vi "Test Basic Messaging.vi"(8 "error in":errorcluster, 11 "Test Case In":refnum<class "Messaging Tests.lvclass">) -> (0 "error out":errorcluster, 3 "Test Case Out":refnum<class "Messaging Tests.lvclass">)   [LabVIEW 2020, in "Messaging Tests.lvlib" / "Messaging Tests.lvclass"]
uses:
  Messaging Tests.lvclass
  C:/Program Files/National Instruments/LabVIEW 2024/vi.lib/Astemes/LUnit/Test Case.lvclass
  TestActor/TestActor.lvclass
  C:/Users/J63553/Projects/_LabVIEW Community/actor-framework/Core/ActorFramework/Actor/Actor.lvclass
  Core/ActorFramework/LastAck/Last Ack.lvclass
  Core/ActorFramework/Message Queue/Message Queue.lvclass/Message Queue.ctl
  Increment Msg/Increment Msg.lvclass/Increment Msg.ctl
  Core/ActorFramework/Message Enqueuer/Message Enqueuer.lvclass/Message Enqueuer.ctl
  Core/ActorFramework/Message Dequeuer/Message Dequeuer.lvclass/Message Dequeuer.ctl
  Core/ActorFramework/LastAck/Last Ack.lvclass/Last Ack.ctl
  TestActor/TestActor.lvclass/TestActor.ctl
  <vilib>/Astemes/LUnit/Test Case.lvclass/Test Case.ctl
  4635b618-f356-4e6f-9d02-cf2597439e9c.vi
  40d5848f-1082-4b1b-baa8-dc5717502d9b.vi
  <vilib>/Astemes/LUnit/Append Pass Result.vi
  <vilib>/Astemes/LUnit/Append Fail Result.vi
  4635b618-f356-4e6f-9d02-cf2597439e9c.vi/9c5d11cd-9439-4240-a1ee-d9baace9c924.vi
  40d5848f-1082-4b1b-baa8-dc5717502d9b.vi/9c5d11cd-9439-4240-a1ee-d9baace9c924.vi
  Core/ActorFramework/Message Enqueuer/Enqueue.vi
  <vilib>/Astemes/LUnit/Run In UI.vi
  <vilib>/Utility/error.llb/Clear Errors.vi
  Increment Msg/Increment Msg.lvclass
  C:/Users/J63553/Projects/_LabVIEW Community/actor-framework/Core/ActorFramework/Message/Message.lvclass
  Core/ActorFramework/Stop Msg/Stop Msg.lvclass
  Core/ActorFramework/Message Priority Queue/Priority Dequeue.vi
  Core/ActorFramework/Message Priority Queue/Priority Enqueue.vi
  Core/ActorFramework/Actor/Actor.lvclass
  Core/ActorFramework/Message Queue/Message Queue.lvclass
  Core/ActorFramework/Message Dequeuer/Message Dequeuer.lvclass
  <vilib>/Astemes/LUnit/Test Case.lvclass
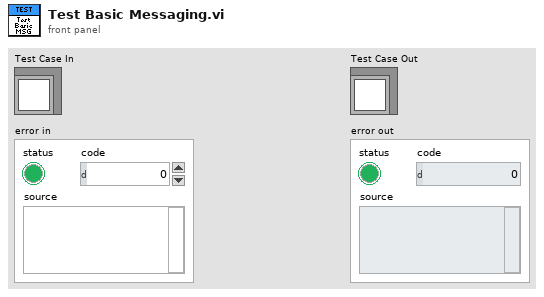
[diagram p1: front panel]
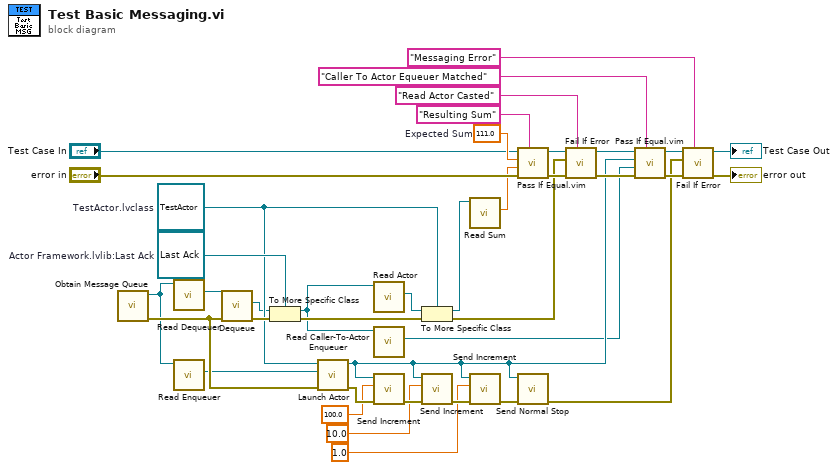
[diagram p0: block diagram]
diagram:
  w13 = 111.0  # Expected Sum
  w22 = refnum<class "Last Ack.lvclass"> refnum  # Actor Framework.lvlib:Last Ack
  w20 = refnum<class "TestActor.lvclass"> refnum  # TestActor.lvclass
  n1 = call "Obtain Message Queue.vi"() -> ("error out"=w34:errorcluster, "Message Queue"=w17:refnum<class "Message Queue.lvclass">)  [unwired: 10 in]
  n2 = call "Read Dequeuer.vi"("Message Queue"=w17) -> ("Message Dequeuer"=w16:refnum<class "Message Dequeuer.lvclass">)  [unwired: 10 in]
  n3 = call "Read Enqueuer.vi"("Message Queue"=w17) -> ("Message Enqueuer"=w18:refnum<class "Message Enqueuer.lvclass">)  [unwired: 10 in]
  n4 = call "Dequeue.vi"("error in (no error)"=w34, "Message Dequeuer in"=w16) -> ("error out"=w33:errorcluster, "Message"=w15:refnum<class "Message.lvclass">)  [unwired: 5 in, 3 out]
  n5 = To More Specific Class(target class=w22, reference=w15, error in=w33) -> (specific class reference=w14:refnum<class "Last Ack.lvclass">, error out=w35:errorcluster)
  n6 = call "Launch Actor.vi"("error in (no error)"=w34, "Actor-to-Caller Enqueuer"=w18, "Actor"=w20) -> ("error out"=w39:errorcluster, "Caller-To-Actor Enqueuer"=w6:refnum<class "Message Enqueuer.lvclass">)  [unwired: 7 in]
  n7 = call "Read Actor.vi"("Last Ack"=w14) -> ("Actor"=w21:refnum<class "Actor.lvclass">)  [unwired: 10 in]
  n8 = call "Read Caller-To-Actor Enqueuer.vi"("Last Ack"=w14) -> ("Caller-to-Actor Enqueuer"=w5:refnum<class "Message Enqueuer.lvclass">)  [unwired: 10 in]
  n9 = call "Send Increment.vi"("error in (no error)"=w39, "Numeric"=100.0, "Actor Framework.lvlib:Send Queue"=w6) -> ("error out"=w38:errorcluster)  [unwired: 8 in]
  n10 = To More Specific Class(target class=w20, reference=w21, error in=w35) -> (specific class reference=w19:refnum<class "TestActor.lvclass">, error out=w31:errorcluster)
  n11 = call "Send Increment.vi"("error in (no error)"=w38, "Numeric"=10.0, "Actor Framework.lvlib:Send Queue"=w6) -> ("error out"=w37:errorcluster)  [unwired: 8 in]
  n12 = call "Read Sum.vi"("TestActor in"=w19) -> ("Sum"=w12:dbl)  [unwired: 9 in, 1 out]
  n13 = call "Send Increment.vi"("error in (no error)"=w37, "Numeric"=1.0, "Actor Framework.lvlib:Send Queue"=w6) -> ("error out"=w36:errorcluster)  [unwired: 8 in]
  n14 = call "Pass If Equal.vim"("Description"="Resulting Sum", "error in (no error)"="error in", "Actual"=w12, "Expected"=w13, "LUnit Test Case In"="Test Case In") -> ("error out"=w32:errorcluster, "LUnit Test Case Out"=w10:refnum<class "Messaging Tests.lvclass">)  [unwired: 5 in]
  n15 = call "Send Normal Stop.vi"("error in (no error)"=w36, "Message Enqueuer"=w6) -> ("error out"=w28:errorcluster)  [unwired: 9 in]
  n16 = call <vilib>:"Fail If Error.vi"("Description"="Read Actor Casted", "error in (no error)"=w32, "Assert error"=w31, "LUnit Test Case In"=w10) -> ("error out"=w29:errorcluster, "LUnit Test Case Out"=w7:refnum<class "Messaging Tests.lvclass">)  [unwired: 6 in]
  n17 = call "Pass If Equal.vim"("Description"="Caller To Actor Equeuer Matched", "error in (no error)"=w29, "Actual"=w5, "Expected"=w6, "LUnit Test Case In"=w7) -> ("error out"=w30:errorcluster, "LUnit Test Case Out"=w8:refnum<class "Messaging Tests.lvclass">)  [unwired: 5 in]
  n18 = call <vilib>:"Fail If Error.vi"("Description"="Messaging Error", "error in (no error)"=w30, "Assert error"=w28, "LUnit Test Case In"=w8) -> ("error out"=→"error out":errorcluster, "LUnit Test Case Out"=→"Test Case Out":refnum<class "Messaging Tests.lvclass">)  [unwired: 6 in]
